vi "NGTS_Select DAQmx Task.vi"(0 "DAQmx Tasks In":refnum<k21>[](array[refnum]), 5 "List of Devices":string[](array[string]), 7 "Type of IO":enum16{"AI", "AO", "DI", "DO"}(ring), 9 "Channel Address":string) -> (4 "DAQmx Tasks Out":refnum<k21>[](array[refnum]), 6 "DAQmx Task Selected Out":refnum<k21>, 10 "index of element":i32)   [LabVIEW 2018]
doc: "Searches the List of Devices for the device specified in the channel address, and returns the corresponding DAQmx task.\n\nBob Hamburger 2008-02-11"
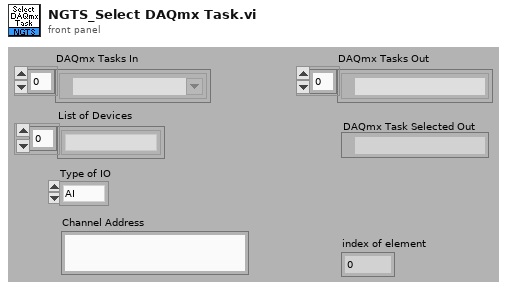
[diagram p1: front panel]
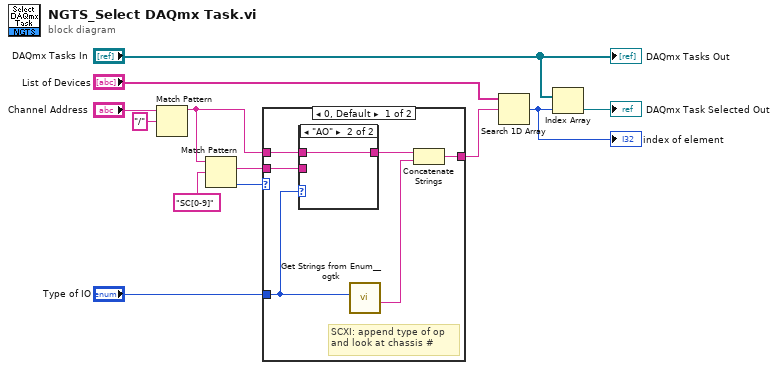
[diagram p0: block diagram]
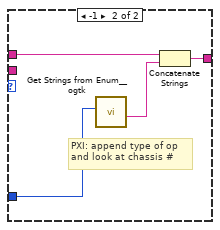
[diagram p3: hidden frame]
diagram:
  n1 = Match Pattern(string="Channel Address", regular expression="/") -> (before substring=w4:string)  [unwired: 1 in, 3 out]
  n2 = Match Pattern(string=w4, regular expression="SC[0-9]") -> (match substring=w2:string, offset past match=w5:i32)  [unwired: 1 in, 2 out]
  n3 = case shown="0, Default" w5 {
    tunnel: w4 -> [w13 w21]
    tunnel: [w17 w22] -> w3
    tunnel: w2 -> [w15 _]
    tunnel: "Type of IO" -> [w16 w24]
    frame 0, Default {
      # "SCXI: append type of op\nand look at chassis #"
      n4 = case shown="\"AO\"" w16 {
        tunnel: [w19 w20] -> w14
        tunnel: w15 -> [w19 _]
        tunnel: w13 -> [_ w20]
        frame "AI", Default {
        }
        frame "AO" {
        }
      }
      n5 = call <userlib>:"Get Strings from Enum__ogtk.vi"("Enum"=w16) -> ("String Value"=w18:string)  [unwired: 7 in, 3 out]
      n6 = Concatenate Strings(w14, w18) -> (w17:string)
    }
    frame -1 {
      # "PXI: append type of op\nand look at chassis #"
      n7 = call <userlib>:"Get Strings from Enum__ogtk.vi"("Enum"=w24) -> ("String Value"=w23:string)  [unwired: 7 in, 3 out]
      n8 = Concatenate Strings(w21, w23) -> (w22:string)
    }
  }
  n9 = Search 1D Array(1D array="List of Devices", element=w3) -> (index of element=w9:i32)  [unwired: 1 in]
  "index of element" <- w9
  n10 = Index Array(array="DAQmx Tasks In", index=w9) -> (element=→"DAQmx Task Selected Out":refnum<k21>)
  "DAQmx Tasks Out" <- "DAQmx Tasks In"
